vi "Knob update positions.vi"(8 "error in":errorcluster, 10 "Keyswitch Cluster":T1, 11 "Knob refference  in":refnum<vi>) -> (0 "error out":errorcluster)   [LabVIEW 2013]
uses:
  KeySwitch Parameters.ctl
  PWM Object Parameters.ctl
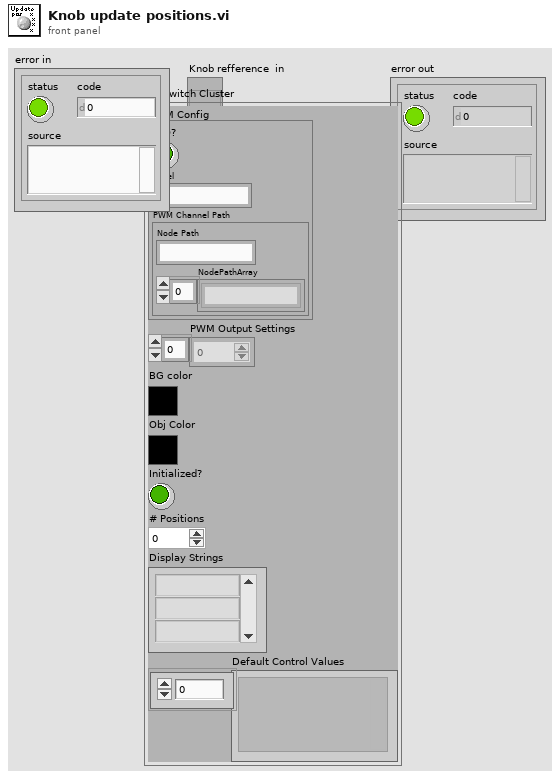
[diagram p1: front panel]
types:
  T1 = typedef "KeySwitch Parameters.ctl" = cluster{"PWM Config":T2, "PWM Output Settings":dbl[], "BG color":u32, "Obj Color":u32, "Initialized?":bool, "# Positions":u8, "Display Strings":string[], "Default Control Values":variant[]}
  T2 = typedef "PWM Object Parameters.ctl" = cluster{"RIO?":bool, "Label":string, "PWM Channel Path":cluster{"NodePathArray":string[], "Node Path":string}}
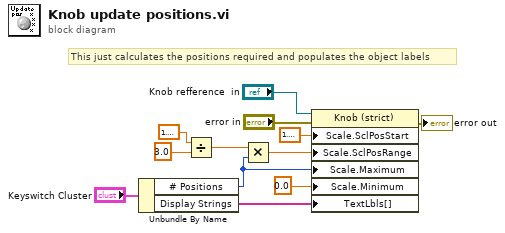
[diagram p0: block diagram]
diagram:
  # "This just calculates the positions required and populates the object labels"
  n1 = Unbundle By Name("Keyswitch Cluster") -> ("# Positions"=w10:u8, "Display Strings"=w12:string[])
  n2 = Divide(x=1.5707963267948966, y=3.0) -> (x/y=w2:dbl)
  n3 = Multiply(x=w2, y=w10) -> (x*y=w4:dbl)
  n4 = property class="Knob (strict)"(reference="Knob refference  in", error in="error in", "Scale.SclPosStart"=1.5707963267948966, "Scale.SclPosRange"=w4, "Scale.Maximum"=w10, "Scale.Minimum"=0.0 ("Scale.Range:Minimum"), "TextLbls[]"=w12) -> (error out=→"error out":errorcluster)  [unwired: 1 out]
